vi "Copy_UI_Data.vi"(8 "error in (no error)":errorcluster, 10 "IB_Source in":refnum<class "IB_Source.lvclass">, 11 "IB_TreeSrcItem.lvclass":refnum<class "IB_Tree_Item_Source.lvclass">) -> (0 "error out":errorcluster, 3 "IB_TreeSrcItem out":refnum<class "IB_Tree_Item_Source.lvclass">)   [LabVIEW 2020, in "IB_Tree_Item_Source.lvclass"]
uses:
  <vilib>/AppBuilder/IB_Classes/Tree_Item_Source/IB_Tree_Item_Source.lvclass
  <vilib>/AppBuilder/IB_Classes/Tree_Item_Source/IB_Tree_Item_Source.lvclass/IB_Tree_Item_Source.ctl
  <vilib>/AppBuilder/IB_Classes/Source/IB_Source.lvclass
  <vilib>/AppBuilder/IB_Classes/Tree_Item/IB_Tree_Item.lvclass
  e:/builds/penguin/labview/branches/2020/dev/dist/vi.lib/AppBuilder/IB_Classes/Tree_Item/IB_Tree_Item.lvclass
  e:/builds/penguin/labview/branches/2020/dev/dist/vi.lib/AppBuilder/IB_Classes/Tree_Item_Source/IB_Tree_Item_Source.lvclass
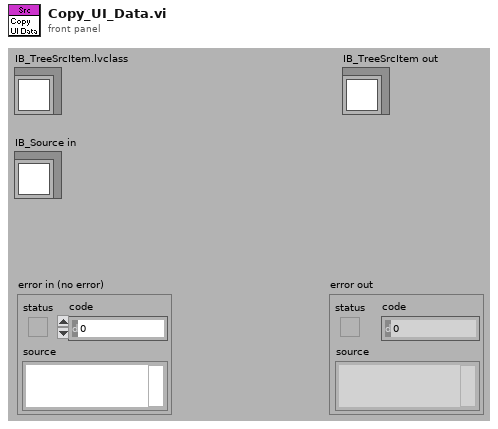
[diagram p1: front panel]
types:
  T1 = typedef "IB_Source.ctl" = cluster{"name":string, "sourceTag":string, "destTag":string, "path":path, "eng_installPath":string, "UI_inBuild?":bool, "str ref?":bool}
  T2 = typedef "IB_Tree_Item.ctl" = cluster{"symbol index":i32, "child tag":string, "parentTag":string, "left cell name":string}
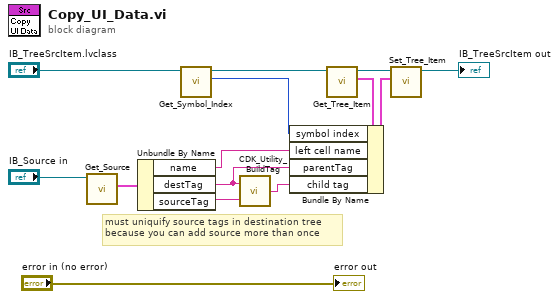
[diagram p0: block diagram]
diagram:
  # "must uniquify source tags in destination tree\nbecause you can add source more than once"
  n1 = call <vilib>:"Get_Source.vi"("IB_Source in"="IB_Source in") -> ("data"=w12:T1)  [unwired: 8 in, 2 out]
  n2 = Unbundle By Name(w12) -> ("name"=w4:string, "destTag"=w10:string, "sourceTag"=w13:string)
  n3 = call-dynamic "Get_Symbol_Index.vi"("IB_TreeItem in"="IB_TreeSrcItem.lvclass") -> ("symbol index"=w1:i32, "IB_TreeItem out"=w2:refnum<class "IB_Tree_Item_Source.lvclass">)  [unwired: 8 in, 1 out]
  n4 = call <resource>:"CDK_Utility_BuildTag.vi"("name or relative path"=w13, "BasePath"=w10) -> ("appended path"=w11:string)
  n5 = call <vilib>:"Get_Tree_Item.vi"("IB_TreeItem in"=w2) -> ("data"=w8:T2, "IB_TreeItem out"=w9:refnum<class "IB_Tree_Item_Source.lvclass">)  [unwired: 8 in, 1 out]
  n6 = Bundle By Name(cluster=w8, "symbol index"=w1, "left cell name"=w4, "parentTag"=w10, "child tag"=w11) -> (w7:T2)
  n7 = call <vilib>:"Set_Tree_Item.vi"("data"=w7, "IB_TreeItem in"=w9) -> ("IB_TreeItem out"=→"IB_TreeSrcItem out":refnum<class "IB_Tree_Item_Source.lvclass">)  [unwired: 8 in, 1 out]
  "error out" <- "error in (no error)"
